vi "FedorReset.vi"(8 "error in (no error)":errorcluster, 10 "DAQmx Device Name":tag="6251") -> (0 "error out":errorcluster)   [LabVIEW 2015]
uses:
  <vilib>/DAQmx/write.llb/DAQmx Write (Digital Bool 1Line 1Point).vi
  <vilib>/DAQmx/create/channels.llb/DAQmx Create Channel (DO-Digital Output).vi
  <vilib>/DAQmx/miscellaneous.llb/DAQmx Fill In Error Info.vi
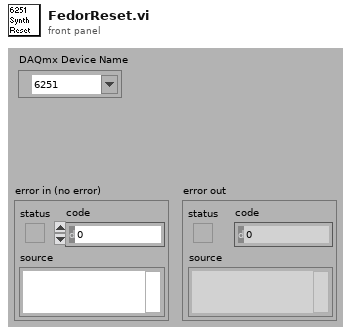
[diagram p1: front panel]
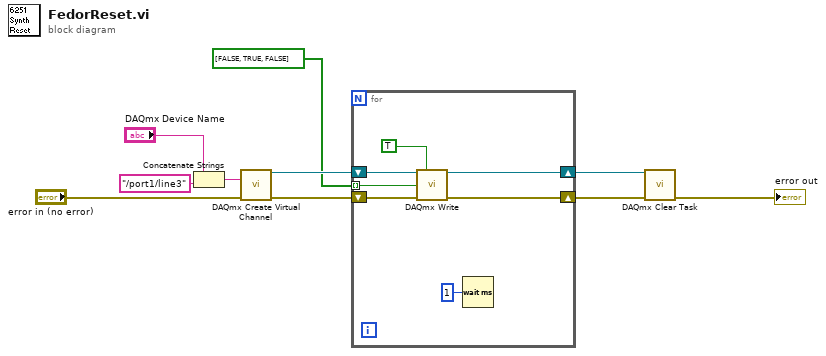
[diagram p0: block diagram]
diagram:
  n1 = Concatenate Strings("DAQmx Device Name", "/port1/line3") -> (w3:string)
  n2 = call-poly <vilib>:"DAQmx Create Virtual Channel.vi"("lines"=w3, "error in"="error in (no error)") -> ("task out"=w9:refnum<k21>, "error out"=w10:errorcluster)  [unwired: 3 in, 9 out]
  n3 = for {
    shift-right: [w15] -> w5
    shift-left: w10 -> [w17]
    shift-right: [w14] -> w8
    shift-left: w9 -> [w16]
    tunnel: bool[] [FALSE, TRUE, FALSE] -> [w11] mode=indexing
    n4 = call-poly <vilib>:"DAQmx Write.vi"("task/channels in"=w16, "auto start"=TRUE, "data"=w11, "error in"=w17) -> ("task out"=w14:refnum<k21>, "error out"=w15:errorcluster)  [unwired: 10 out]
    n5 = Wait (ms)(milliseconds to wait=u32 1) -> ()  [unwired: 1 out]
  }
  n6 = call <vilib>:"DAQmx Clear Task.vi"("task in"=w8, "error in"=w5) -> ("error out"=→"error out":errorcluster)  [unwired: 13 out]
